vi "FuncImg-Parameters.vi"(11 "Error In":errorcluster) -> (15 "Error Out":errorcluster)   [LabVIEW 2020]
uses:
  Typedefs/Functional Parameters Cluster.ctl
  Typedefs/Get-Set-Clear Control.ctl
panel:
  out "File version index (-1 = latest version)":i32
  out "File version index (-1 = latest version)":i32
  out "Norm ROI columns header":string[](array[string])
  out "Normalised ROI file data (header removed)":dbl[][](array[numeric])
  out "Array size":i32[](array[numeric])
  out "File version index (-1 = latest version)":i32
  out "# of ROI":i32
  out "ROI columns header":string[](array[string])
  out "ROI.txt":dbl[][](array[numeric])
  out "Columns header":string[](array[string])
  out "Zplane_Pockels_Values file data (header removed)":dbl[][](array[numeric])
  out "size":i32[](array[numeric])
  # "<--- Z Motor,\t  Z Norm,\t  Laser intensity (a.k.a Pockels)"
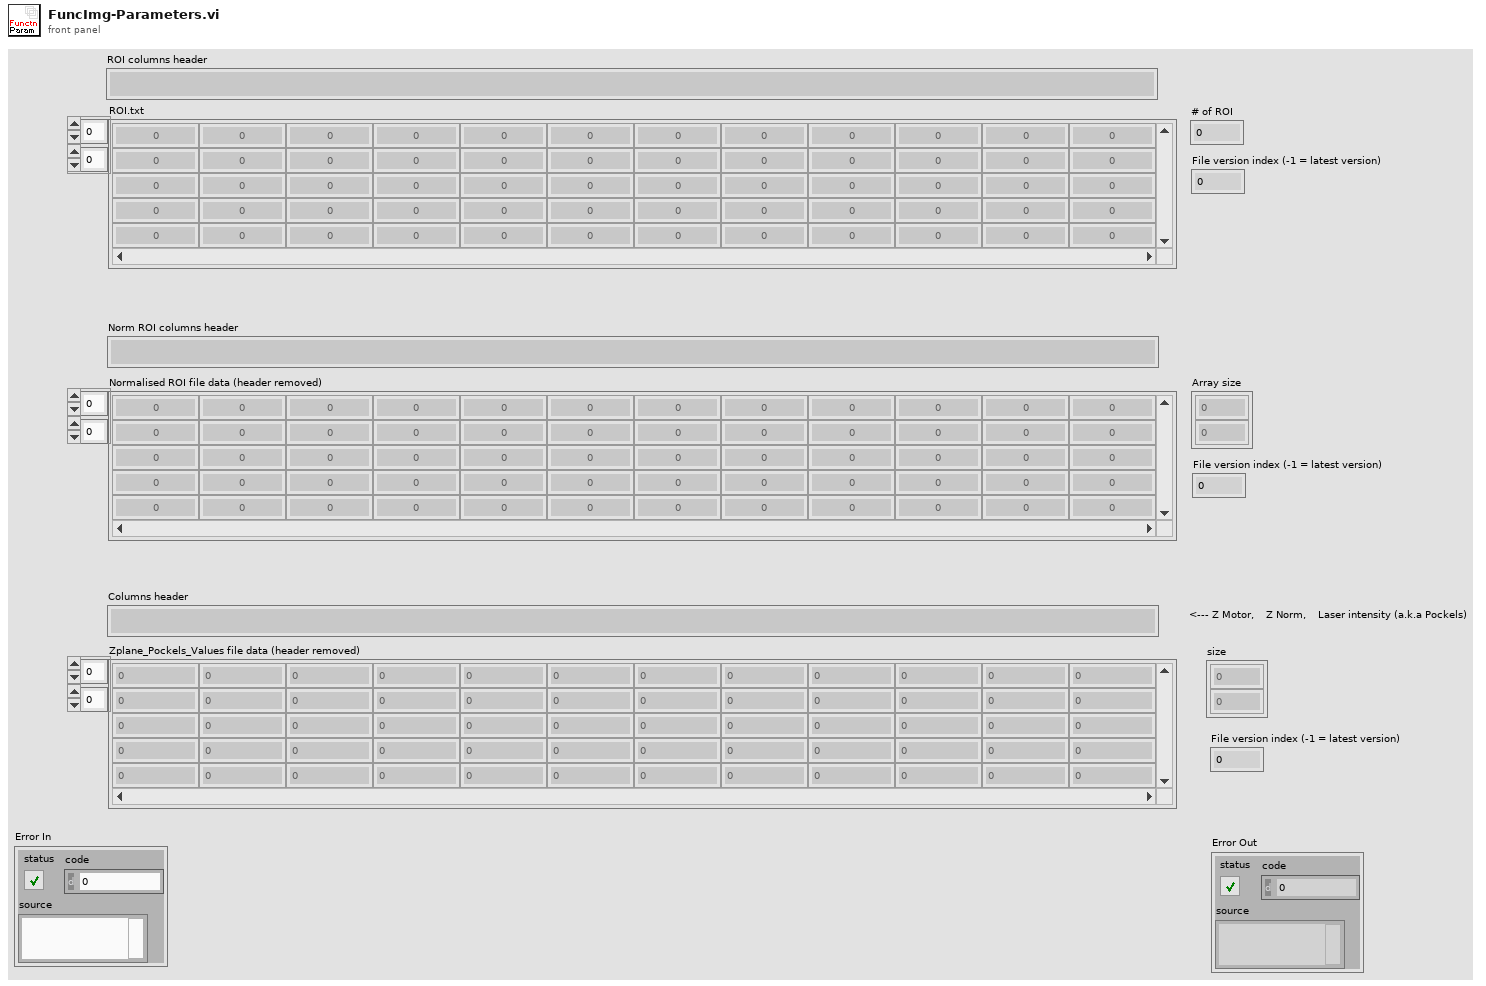
[diagram p1: front panel]
types:
  T1 = typedef "Get-Set-Clear Control.ctl" = enum16{"Get", "Set", "Clear"}
  T2 = typedef "Functional Parameters Cluster.ctl" = cluster{"ROI data":dbl[][], "ROI format version":i32, "Norm ROI data":dbl[][], "Norm. ROI format version":i32, "Z norm":dbl[], "Z norm format version":i32}
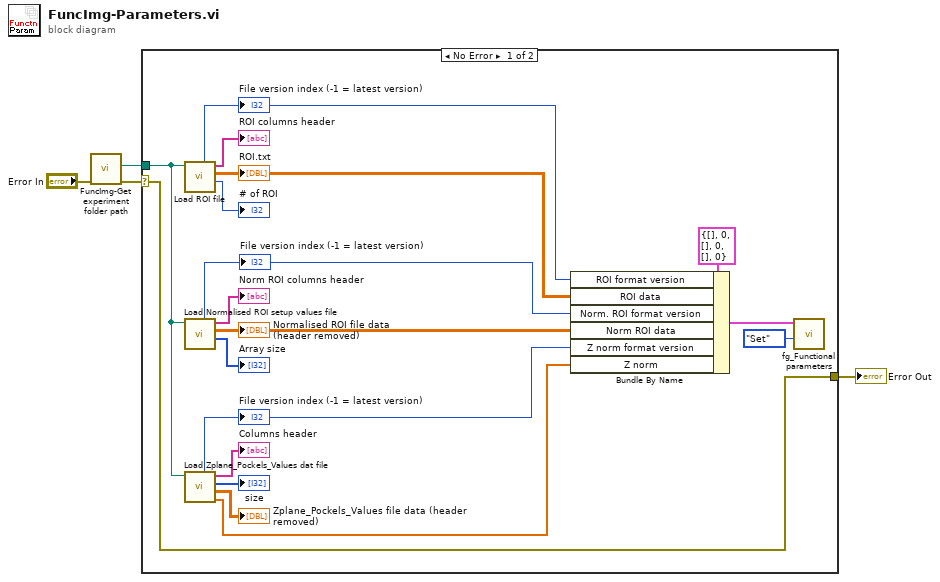
[diagram p0: block diagram]
diagram:
  n1 = call "FuncImg-Get experiment folder path.vi"("error in (no error)"="Error In") -> ("error out"=w2:errorcluster, "Experiment data folder path"=w1:path)  [unwired: 9 in]
  n2 = case shown="No Error" w2 {
    selector: w2 -> [w5 w23]
    tunnel: w1 -> [w11 _]
    tunnel: [w5 w23] -> w4
    frame No Error {
      n3 = call "Load ROI file.vi"("Experiment data folder path"=w11) -> ("Number of ROI"=→"# of ROI":i32, "ROI Data (header removed)"=w13:dbl[][], "ROI columns header"=→"ROI columns header":string[], "Version index (-1 = latest version)"=w10:i32)  [unwired: 7 in]
      "ROI.txt" <- w13
      "File version index (-1 = latest version)" <- w10
      n4 = call "Load Normalised ROI setup values file.vi"("Experiment data folder path"=w11) -> ("Normalised ROI file data size"=→"Array size":i32[], "Normalised ROI file data (header removed)"=w9:dbl[][], "Norm ROI columns header"=→"Norm ROI columns header":string[], "Version index (-1 = latest version)"=w8:i32)  [unwired: 7 in]
      "Normalised ROI file data (header removed)" <- w9
      "File version index (-1 = latest version)" <- w8
      n5 = call "Load Zplane_Pockels_Values dat file.vi"("Experiment data folder path"=w11) -> ("[AOL Z (um)]"=w7:dbl[], "Zplane_Pockels_Values file data (header removed)"=→"Zplane_Pockels_Values file data (header removed)":dbl[][], "2D array size"=→"size":i32[], "Columns header"=→"Columns header":string[], "Version index (-1 = latest version)"=w6:i32)  [unwired: 5 in, 1 out]
      "File version index (-1 = latest version)" <- w6
      n6 = Bundle By Name(cluster=T2 {"ROI data"=[], "ROI format version"=0, "Norm ROI data"=[], "Norm. ROI format version"=0, "Z norm"=[], "Z norm format version"=0} ("Functional Parameters"), "ROI format version"=w10, "ROI data"=w13, "Norm. ROI format version"=w8, "Norm ROI data"=w9, "Z norm format version"=w6, "Z norm"=w7) -> (w21:T2)
      n7 = call "fg_Functional parameters.vi"("Function"=Get-Set-Clear_Control."Set", "Functional Parameters in"=w21) -> ()  [unwired: 6 in, 4 out]
    }
    frame Error {
    }
  }
  "Error Out" <- w4
